vi "Set Optimiser Parameters and Observables.vi"(0 "Optimiser SBlock in":refnum<class "Optimiser SBlock.lvclass">, 5 "Parameters":T3[](array[typedef]), 7 "Parameters - string":T1[](array[typedef]), 9 "Observables":T2[](array[typedef]) {"Weight" min=0.0 max=1.0}, 11 "error in (no error)":errorcluster, 12 "Number of Exploration Runs":i32) -> (4 "Optimiser SBlock out":refnum<class "Optimiser SBlock.lvclass">, 15 "error out":errorcluster)   [LabVIEW 2020, in "CIRCUS_uServices.lvlib" / "Run Utilities.lvlib" / "Optimiser SBlock.lvclass"]
uses:
  Optimiser SBlock.lvclass
  Optimiser Cell/Optimiser Cell.lvclass
  Optimiser Cell/Optimise parameter - numeric.ctl
  Optimiser Cell/Optimisation observable.ctl
  Optimiser Cell/Optimise parameter - string.ctl
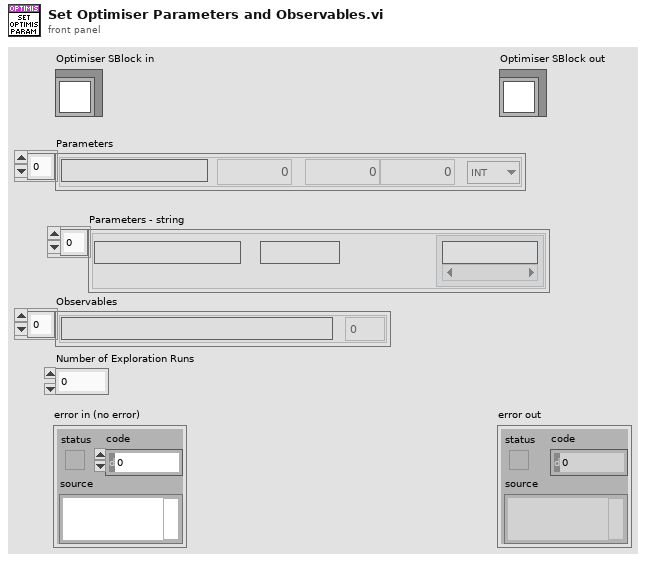
[diagram p1: front panel]
types:
  T1 = typedef "CIRCUS_uServices.lvlib/Run Utilities.lvlib/Optimiser Cell.lvclass/Optimise parameter - string.ctl" = cluster{"Name":string, "Start value":string, "Options":string[]}
  T2 = typedef "CIRCUS_uServices.lvlib/Run Utilities.lvlib/Optimiser Cell.lvclass/Optimisation observable.ctl" = cluster{"Name":string, "Weight":dbl}
  T3 = typedef "CIRCUS_uServices.lvlib/Run Utilities.lvlib/Optimiser Cell.lvclass/Optimise parameter - numeric.ctl" = cluster{"Name":string, "Start value":dbl, "From":dbl, "To":dbl, "dtype":enum16{"INT", "DBL"}}
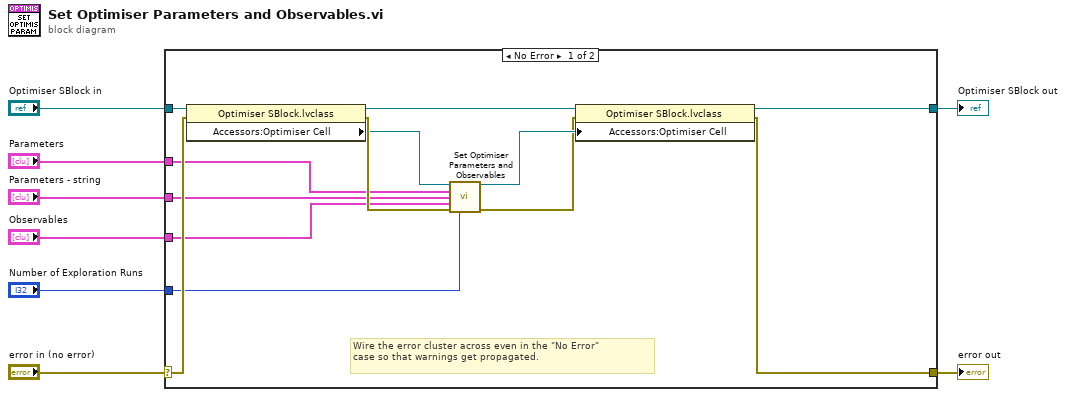
[diagram p0: block diagram]
diagram:
  n1 = case shown="No Error" "error in (no error)" {
    selector: "error in (no error)" -> [w15 w23]
    tunnel: [w16 w23] -> w7
    tunnel: [w17 w22] -> w5
    tunnel: "Optimiser SBlock in" -> [w20 w22]
    tunnel: "Parameters" -> [w14 _]
    tunnel: "Observables" -> [w13 _]
    tunnel: "Parameters - string" -> [w10 _]
    tunnel: "Number of Exploration Runs" -> [w9 _]
    frame No Error {
      # "Wire the error cluster across even in the \"No Error\"\ncase so that warnings get propagated."
      n2 = property class="Optimiser SBlock.lvclass"(reference=w20, error in=w15) -> (reference out=w18:refnum<class "Optimiser SBlock.lvclass">, error out=w21:errorcluster, "Accessors:Optimiser Cell"=w19:refnum<class "Optimiser Cell.lvclass">)
      n3 = call-dynamic "Set Optimiser Parameters and Observables.vi"("Optimiser Cell in"=w19, "Parameters"=w14, "Parameters - string"=w10, "Observables"=w13, "error in (no error)"=w21, "Number of Exploration Runs"=w9) -> ("Optimiser Cell out"=w12:refnum<class "Optimiser Cell.lvclass">, "error out"=w11:errorcluster)  [unwired: 8 in]
      n4 = property class="Optimiser SBlock.lvclass"(reference=w18, error in=w11, "Accessors:Optimiser Cell"=w12) -> (reference out=w17:refnum<class "Optimiser SBlock.lvclass">, error out=w16:errorcluster)
    }
    frame Error {
    }
  }
  "error out" <- w7
  "Optimiser SBlock out" <- w5
